vi "Engine-RPC-PWMPumpB.vi"(8 "Error In":errorcluster, 11 "DSI Reference":refnum<class "DCM-DSI.lvclass">) -> (0 "Error Out":errorcluster, 3 "DSI Reference":refnum<class "DCM-DSI.lvclass">)   [LabVIEW 2016, in "DSI-RT.lvlib"]
uses:
  DSI-RT.lvlib
  Classes/DCM-DSI/DCM-DSI.lvclass
  <vilib>/Powertrain Controls/Device Drivers/DCM/HH/FPGA/Mode.ctl
  <vilib>/Powertrain Controls/Device Drivers/DCM/HH/RT/Setup.ctl
  <vilib>/Powertrain Controls/Device Drivers/DCM/Rev0/FPGA/Digital Channel.ctl
  <vilib>/Powertrain Controls/Device Drivers/DCM/HH/RT/Angle Control.ctl
  <vilib>/Powertrain Controls/Device Drivers/DCM/Rev0/RT/DCM - RT.lvclass/DCM - RT.ctl
  <vilib>/Powertrain Controls/Device Drivers/DCM/HH/RT/Mode.ctl
  <vilib>/addons/Software Calibration Management/xSCM/Controls/TBL1D.ctl
  <vilib>/Powertrain Controls/Device Drivers/DCM/Rev0/RT/Read HH Mode.vi
  Classes/DCM-DSI/Read HH Command.vi
  Classes/DCM-DSI/Read Channels.vi
  Classes/DCM-DSI/Read dt.vi
  Classes/DCM-DSI/Read System ADC.vi
  Classes/DCM-DSI/Read DCM Ref.vi
  Classes/DCM-DSI/Write HH Command.vi
  <vilib>/Powertrain Controls/Device Drivers/DCM/Rev0/RT/DCM - RT.lvclass
  <vilib>/addons/Software Calibration Management/xSCM/CalPoint.xnode
  <vilib>/addons/Software Calibration Management/xSCM/FaultPoint.xnode
  <vilib>/Powertrain Controls/Device Drivers/DCM/HH/FPGA/DCM - FPGA - HH.lvlib
  <vilib>/addons/Software Calibration Management/xSCM/ni_scm.dll
  <vilib>/addons/Software Calibration Management/xSCM/SCM-API.lvlib
  <vilib>/Powertrain Controls/Device Drivers/DCM/HH/RT/DCM - RT - HH.lvlib
  <vilib>/Powertrain Controls/Device Drivers/DCM/Rev0/FPGA/DCM - FPGA.lvlib
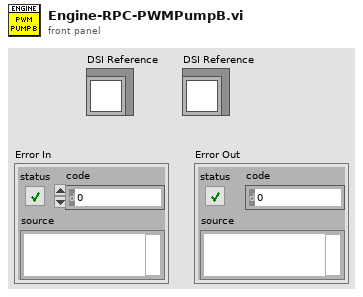
[diagram p1: front panel]
types:
  T1 = typedef "DCM - RT - HH.lvlib/Setup.ctl" = cluster{"Mode":T2, "Digital Input":T3, "Polarity":bool, "Frequency [Hz]":sgl, "Duty Cycle [%]":sgl, "TDC Offset [CAD]":sgl, "Window Start [DBTDC]":sgl, "Window End [DBTDC]":sgl, "Angles":T4[], "Skip Fire":bool, "Skip Fire Index":u8}
  T2 = typedef "DCM - FPGA - HH.lvlib/Mode.ctl" = enum8{"Off", "Direct", "Pulse Width Modulation", "Engine Position Tracking"}
  T3 = typedef "DCM - FPGA.lvlib/Digital Channel.ctl" = enum8{"Unused", "User OS", "Diff IO 1", "Diff IO 2", "Diff IO 3", "Diff IO 4", "Diff IO 5", "Diff IO 6", "Diff IO 7", "Diff IO 8", "Aux 1", "Aux 2", "Aux 3", "Aux 4", "Aux 5", "Aux 6", "Aux 7", "Aux 8", "Aux 9", "Aux 10", "Aux 11", "Aux 12", "Aux 13", "Aux 14", "Aux 15", "Aux 16"}
  T4 = typedef "DCM - RT - HH.lvlib/Angle Control.ctl" = cluster{"Enable":bool, "Location [DBTDC]":sgl, "Duration [s]":sgl}
  T5 = cluster{"IMV":cluster{"Current_Calc":sgl, "DutyCyc_PIDOut":sgl, "DutyCyc_MaxCalc":sgl, "DutyCyc_Des":sgl}, "HPV":cluster{"Current_Calc":sgl, "DutyCyc_TblOut":sgl, "DutyCyc_MaxCalc":sgl, "DutyCyc_Des":sgl}}
  T6 = cluster{"PID_Kp":sgl, "PID_Ti":sgl, "PID_Td":sgl, "PID_FF":sgl, "Non-PID_FF":sgl, "PID_Min":sgl, "PID_Max":sgl}
  T7 = typedef "DCM-DSI.lvclass/Channel.ctl" = cluster{"Name":string, "Unit":string, "Value":sgl}
  T8 = typedef "DCM - RT.lvclass/System ADC.ctl" = cluster{"AI 1 [V]":sgl, "AI 2 [V]":sgl, "AI 3 [V]":sgl, "AI 4 [V]":sgl, "AI 5 [V]":sgl, "AI 6 [V]":sgl, "AI 7 [V]":sgl, "AI 8 [V]":sgl, "AI 9 [V]":sgl, "AI 10 [V]":sgl, "AI 11 [V]":sgl, "AI 12 [V]":sgl, "Temp HH 1-6 [C]":sgl, "Temp HH 7-12 [C]":sgl, "Temp DI A [C]":sgl, "Temp DI Zener A [C]":sgl, "Temp DI B [C]":sgl, "Temp DI Zener B [C]":sgl, "Temp CPU [C]":sgl, "Temp Fan Intake [C]":sgl, "Temp Secondary A [C]":sgl, "Temp Primary A [C]":sgl, "Temp Boost B [C]":sgl, "Primary Range [V]":sgl, "Primary A1A2 [V]":sgl, "Primary A3A4 [V]":sgl, "Primary B3B4 [V]":sgl, "Primary B1B2 [V]":sgl, "Secondary A1A2 [V]":sgl, "Secondary A3A4 [V]":sgl, "Secondary B3B4 [V]":sgl, "Secondary B1B2 [V]":sgl, "Ext HV A [V]":sgl, "Ext HV B [V]":sgl, "FET Driver [V]":sgl, "Fan [V]":sgl, "Battery [V]":sgl, "DRVP [V]":sgl, "Key [V]":sgl, "DI Zener A [V]":sgl, "DI Zener B [V]":sgl, "Pump Zener A [V]":sgl, "Pump Zener B [V]":sgl, "MPRD [V]":sgl}
  T9 = typedef "DCM - RT - HH.lvlib/Mode.ctl" = enum16{"Off", "Lowside", "Highside", "PFI", "Full H", "3-Phase"}
  T10 = cluster{"IMV":cluster{"PWMFreq":sgl, "NomResistance":sgl, "DutyCyc_Max":sgl, "Min Duty Cycle":sgl, "DutyCycle_ManE":bool, "DutyCycle_Man":sgl}, "HPV":cluster{"PWMFreq":sgl, "NomResistance":sgl, "DutyCyc_Max":sgl, "Min Duty Cycle":sgl, "DutyCycle_ManE":bool, "DutyCycle_Man":sgl}}
  T11 = typedef "SCM-API.lvlib/TBL1D.ctl" = cluster{"X":sgl[], "Y":sgl[]}
  T12 = cluster{"PWMFreq":sgl, "NomResistance":sgl, "DutyCyc_Max":sgl, "Min Duty Cycle":sgl, "DutyCycle_ManE":bool, "DutyCycle_Man":sgl}
  T13 = cluster{"Current_Calc":sgl, "DutyCyc_PIDOut":sgl, "DutyCyc_MaxCalc":sgl, "DutyCyc_Des":sgl}
  T14 = cluster{"ProportionalAction":sgl, "IntegralAction":sgl, "DerivativeAction":sgl}
  T15 = cluster{"Enable LS Channel":bool, "Freq [Hz]":sgl, "DutyCyc [%]":sgl}
  T16 = cluster{"Current_Calc":sgl, "DutyCyc_TblOut":sgl, "DutyCyc_MaxCalc":sgl, "DutyCyc_Des":sgl}
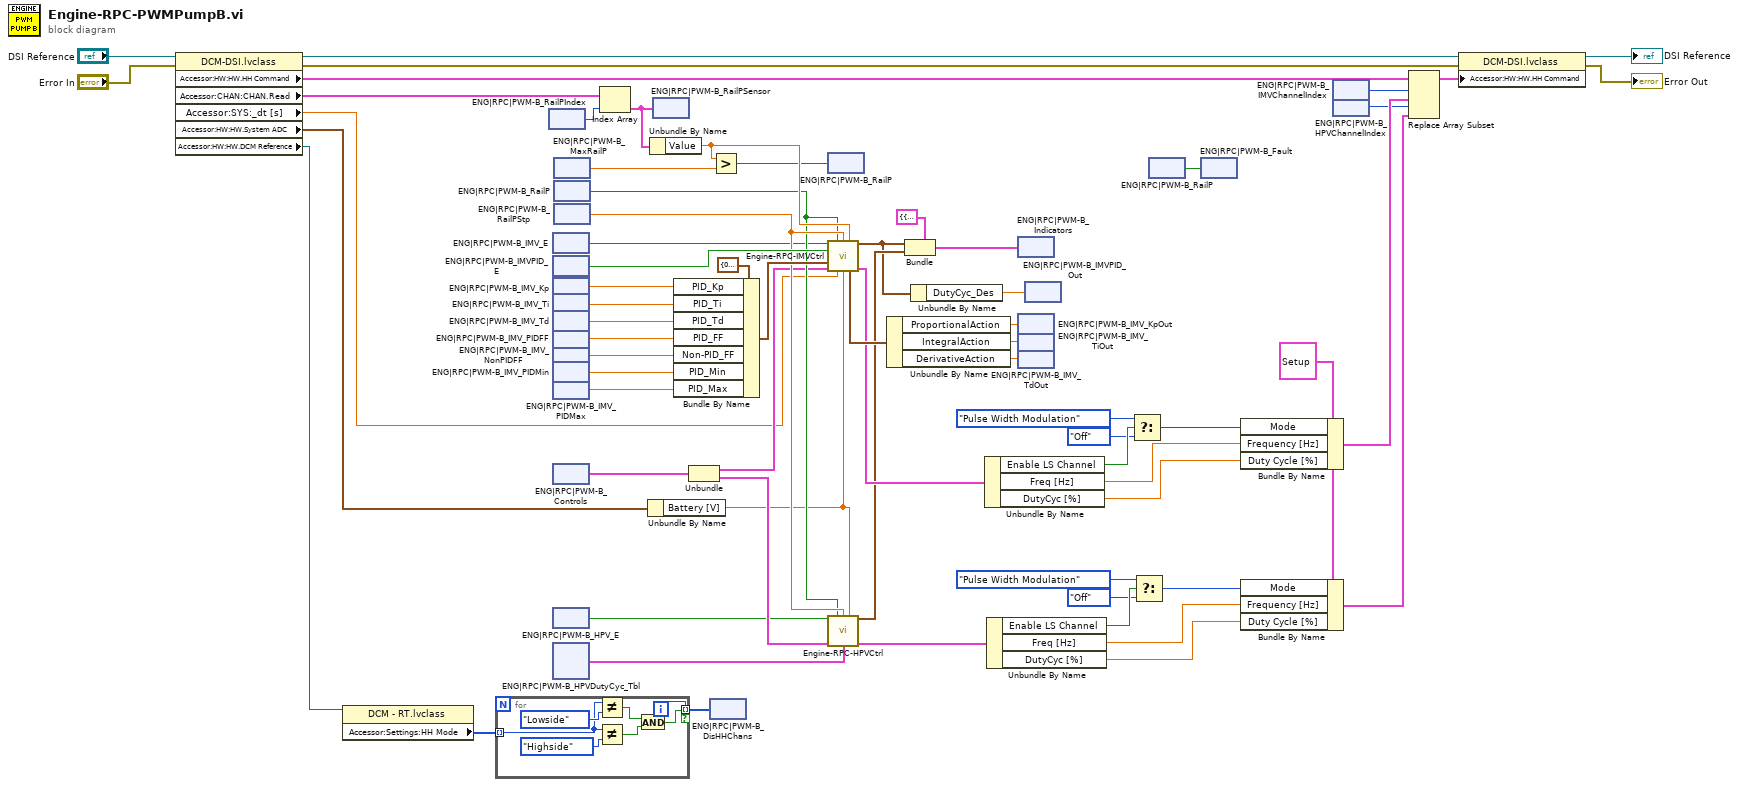
[diagram p0: block diagram]
diagram:
  w15 = T1 {"Mode"=enum."Off", "Digital Input"=enum."Unused", "Polarity"=FALSE, "Frequency [Hz]"=0.0, "Duty Cycle [%]"=0.0, "TDC Offset [CAD]"=0.0, "Window Start [DBTDC]"=0.0, "Window End [DBTDC]"=0.0, "Angles"=[], "Skip Fire"=FALSE, "Skip Fire Index"=0} ("HH Command")
  n1 = property class="DCM-DSI.lvclass"(reference="DSI Reference", error in="Error In") -> (reference out=w19:refnum<class "DCM-DSI.lvclass">, error out=w18:errorcluster, "Accessor:HW:HW.HH Command"=w14:T1[], "Accessor:CHAN:CHAN.Read"=w3:T7[], "Accessor:SYS:_dt [s]"=w5:sgl, "Accessor:HW:HW.System ADC"=w6:T8, "Accessor:HW:HW.DCM Reference"=w4:refnum<class "DCM - RT.lvclass">)
  n2 = property class="DCM - RT.lvclass"(reference=w4) -> ("Accessor:Settings:HH Mode"=w8:T9[])  [unwired: 1 in, 2 out]
  n3 = for {
    tunnel: [w73] -> w7 mode=indexing if=w71
    tunnel: w8 -> [w68] mode=indexing
    i -> [w73]
    n4 = Not Equal?(x=w68, y=Mode."Lowside" ("Mode")) -> (x != y?=w70:bool)
    n5 = Not Equal?(x=w68, y=Mode."Highside" ("Mode")) -> (x != y?=w69:bool)
    n6 = And(x=w70, y=w69) -> (x .and. y?=w71:bool)
  }
  n7 = xnode "ENG|RPC|PWM-B_RailPIndex"() -> ("Value"=w2:i32)
  n8 = xnode "ENG|RPC|PWM-B_IMV_E"() -> ("Value"=w29:bool)
  n9 = xnode "ENG|RPC|PWM-B_IMVPID_E"() -> ("Value"=w41:bool)
  n10 = xnode "ENG|RPC|PWM-B_IMV_Kp"() -> ("Value"=w55:sgl)
  n11 = xnode "ENG|RPC|PWM-B_IMV_Ti"() -> ("Value"=w56:sgl)
  n12 = xnode "ENG|RPC|PWM-B_IMV_Td"() -> ("Value"=w57:sgl)
  n13 = xnode "ENG|RPC|PWM-B_IMV_PIDFF"() -> ("Value"=w58:sgl)
  n14 = xnode "ENG|RPC|PWM-B_IMV_NonPIDFF"() -> ("Value"=w59:sgl)
  n15 = xnode "ENG|RPC|PWM-B_IMV_PIDMin"() -> ("Value"=w60:sgl)
  n16 = xnode "ENG|RPC|PWM-B_IMV_PIDMax"() -> ("Value"=w61:sgl)
  n17 = xnode "ENG|RPC|PWM-B_Controls"() -> ("Value"=w28:T10)
  n18 = xnode "ENG|RPC|PWM-B_HPV_E"() -> ("Value"=w23:bool)
  n19 = xnode "ENG|RPC|PWM-B_HPVDutyCyc_Tbl"() -> ("Value"=w24:T11)
  n20 = xnode "ENG|RPC|PWM-B_MaxRailP"() -> ("Value"=w38:sgl)
  n21 = xnode "ENG|RPC|PWM-B_RailP"() -> ("Fault"=w36:bool)
  n22 = xnode "ENG|RPC|PWM-B_RailPStp"() -> ("Value"=w40:sgl)
  n23 = Index Array(array=w3, index=w2) -> (element=w1:T7)
  n24 = Unbundle By Name(w6) -> ("Battery [V]"=w25:sgl)
  n25 = Unbundle By Name(w1) -> ("Value"=w39:sgl)
  n26 = xnode "ENG|RPC|PWM-B_RailPSensor"("Value"=w1) -> ()
  n27 = Bundle By Name(cluster=T6 {"PID_Kp"=0.0, "PID_Ti"=0.01, "PID_Td"=0.0, "PID_FF"=0.0, "Non-PID_FF"=0.0, "PID_Min"=-100.0, "PID_Max"=100.0} ("PID Settings"), "PID_Kp"=w55, "PID_Ti"=w56, "PID_Td"=w57, "PID_FF"=w58, "Non-PID_FF"=w59, "PID_Min"=w60, "PID_Max"=w61) -> (w43:T6)
  n28 = Unbundle(w28) -> ("IMV"=w27:T12, "HPV"=w26:T12)
  n29 = xnode "ENG|RPC|PWM-B_DisHHChans"("Value"=w7) -> ()
  n30 = Greater?(x=w39, y=w38) -> (0:w37:bool)
  n31 = xnode "ENG|RPC|PWM-B_RailP"("Fault"=w37) -> ()
  n32 = call "Engine-RPC-IMVCtrl.vi"("Control Enable"=w29, "Fault Input"=w36, "Rail Press Setpoint"=w40, "Rail Pressure"=w39, "PID Enable"=w41, "PID Settings"=w43, "Output Management Controls"=w27, "dt (s)"=w5, "Battery [V]"=w25) -> ("Output"=w22:T13, "PID_Action_Output"=w65:T14, "LS Output"=w48:T15)  [unwired: 4 in]
  n33 = call "Engine-RPC-HPVCtrl.vi"("Control Enable"=w23, "Fault Input"=w36, "RailP Setpoint"=w40, "Battery [V]"=w25, "Output Management Controls"=w26, "Open Loop DC Table"=w24) -> ("Output"=w31:T16, "LS Output"=w42:T15)  [unwired: 8 in]
  n34 = Unbundle By Name(w65) -> ("ProportionalAction"=w64:sgl, "IntegralAction"=w63:sgl, "DerivativeAction"=w62:sgl)
  n35 = Bundle(cluster=T5 {"IMV"={"Current_Calc"=0.0, "DutyCyc_PIDOut"=0.0, "DutyCyc_MaxCalc"=0.0, "DutyCyc_Des"=0.0}, "HPV"={"Current_Calc"=0.0, "DutyCyc_TblOut"=0.0, "DutyCyc_MaxCalc"=0.0, "DutyCyc_Des"=0.0}} ("Value"), "IMV"=w22, "HPV"=w31) -> (w30:T5)
  n36 = Unbundle By Name(w22) -> ("DutyCyc_Des"=w21:sgl)
  n37 = Unbundle By Name(w48) -> ("Enable LS Channel"=w53:bool, "Freq [Hz]"=w51:sgl, "DutyCyc [%]"=w50:sgl)
  n38 = Unbundle By Name(w42) -> ("Enable LS Channel"=w49:bool, "Freq [Hz]"=w34:sgl, "DutyCyc [%]"=w33:sgl)
  n39 = xnode "ENG|RPC|PWM-B_Indicators"("Value"=w30) -> ()
  n40 = xnode "ENG|RPC|PWM-B_IMV_KpOut"("Value"=w64) -> ()
  n41 = xnode "ENG|RPC|PWM-B_IMV_TiOut"("Value"=w63) -> ()
  n42 = xnode "ENG|RPC|PWM-B_IMV_TdOut"("Value"=w62) -> ()
  n43 = xnode "ENG|RPC|PWM-B_IMVPID_Out"("Value"=w21) -> ()
  n44 = Select(t=Mode."Pulse Width Modulation" ("Mode"), s=w53, f=Mode."Off" ("Mode")) -> (s? t:f=w52:T2)
  n45 = Select(t=Mode."Pulse Width Modulation" ("Mode"), s=w49, f=Mode."Off" ("Mode")) -> (s? t:f=w35:T2)
  n46 = xnode "ENG|RPC|PWM-B_RailP"() -> ("Fault"=w20:bool)
  n47 = xnode "ENG|RPC|PWM-B_Fault"("Value"=w20) -> ()
  n48 = Bundle By Name(cluster=w15, "Mode"=w52, "Frequency [Hz]"=w51, "Duty Cycle [%]"=w50) -> (w11:T1)
  n49 = Bundle By Name(cluster=w15, "Mode"=w35, "Frequency [Hz]"=w34, "Duty Cycle [%]"=w33) -> (w12:T1)
  n50 = xnode "ENG|RPC|PWM-B_IMVChannelIndex"() -> ("Value"=w10:i32)
  n51 = xnode "ENG|RPC|PWM-B_HPVChannelIndex"() -> ("Value"=w9:i32)
  n52 = Replace Array Subset(array=w14, new element #1=w11, index #1=w10, new element #2=w12, index #2=w9) -> (w13:T1[])
  n53 = property class="DCM-DSI.lvclass"(reference=w19, error in=w18, "Accessor:HW:HW.HH Command"=w13) -> (reference out=→"DSI Reference":refnum<class "DCM-DSI.lvclass">, error out=→"Error Out":errorcluster)
